vi "AccelerometerEventExe.vi"(0 "Devices In":u64[](array[numeric]), 5 "Event Registration Refnum In":refnum<event-registration>, 11 "error in (no error)":errorcluster) -> (2 "Index":i32, 3 "Event?":bool, 4 "Devices Out":u64[](array[numeric]), 6 "Event Registration Refnum Out":refnum<event-registration>, 8 "Accel Data":dbl[](array[numeric]), 10 "Timestamp":dbl, 14 "phid":u64, 15 "error out":errorcluster)   [LabVIEW 2020, in "Phidget Accelerometer.lvlib"]
doc: "${AccelerationChange:Header}"
uses:
  <instrlib>/Phidgets/Phidget Accelerometer/Phidget Accelerometer.lvlib
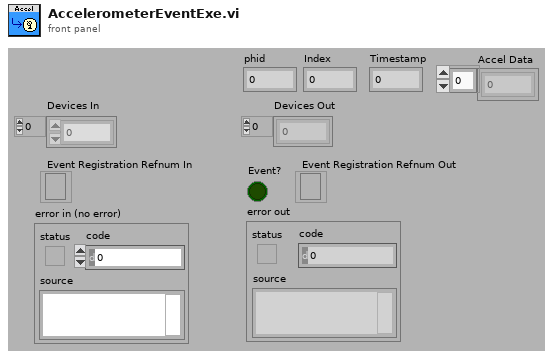
[diagram p1: front panel]
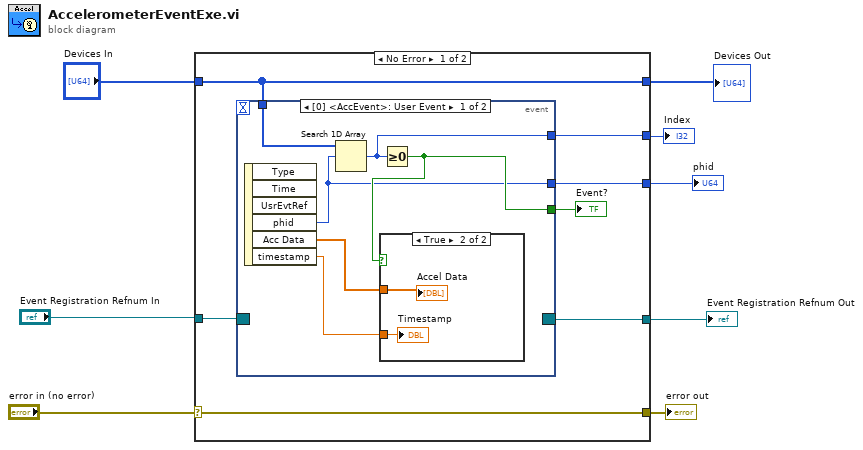
[diagram p0: block diagram]
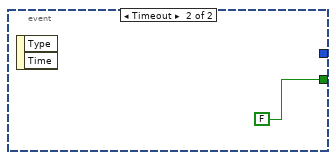
[diagram p3: hidden frame]
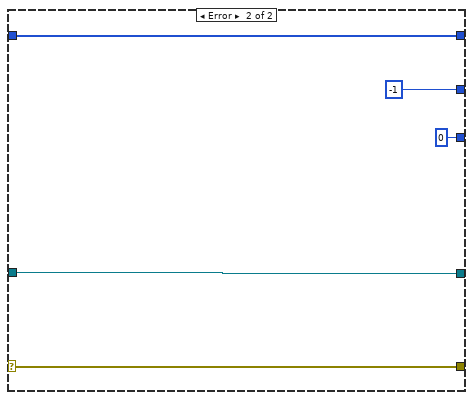
[diagram p4: hidden frame]
diagram:
  n1 = case shown="No Error" "error in (no error)" {
    selector: "error in (no error)" -> [w12 w29]
    tunnel: [w12 w29] -> w7
    tunnel: [w15 w28] -> w2
    tunnel: "Event Registration Refnum In" -> [w14 w28]
    tunnel: [w11 w27] -> w5
    tunnel: "Devices In" -> [w11 w27]
    tunnel: [w10 -1] -> w4
    tunnel: [w9 u64 0 ("phid")] -> w3
    frame No Error {
      n2 = event shown="[0] <AccEvent>: User Event" {
        selector: w14 -> [_ _]
        dyn-events: [_ _] -> w15
        timeout: _ -> [_ _]
        tunnel: [w20 FALSE] -> w13
        tunnel: w11 -> [w21 _]
        tunnel: [w19 _] -> w10
        tunnel: [w17 _] -> w9
        event User Event {
          n3 = event-data() -> ("phid"=w17:u64, "Acc Data"=w16:dbl[], "timestamp"=w18:dbl)  [unwired: 1 in, 3 out]
          n4 = Search 1D Array(1D array=w21, element=w17) -> (index of element=w19:i32)  [unwired: 1 in]
          n5 = Greater Or Equal To 0?(x=w19) -> (x >= 0?=w20:bool)
          n6 = case shown="True" w20 {
            tunnel: w16 -> [_ w23]
            tunnel: w18 -> [_ w22]
            frame False {
            }
            frame True {
              "Accel Data" <- w23
              "Timestamp" <- w22
            }
          }
        }
        event Timeout {
          n7 = event-data() -> ()  [unwired: 1 in, 2 out]
        }
      }
      "Event?" <- w13
    }
    frame Error {
    }
  }
  "error out" <- w7
  "Devices Out" <- w5
  "Index" <- w4
  "phid" <- w3
  "Event Registration Refnum Out" <- w2
